vi "ROS_Dummy_Test.vi"() -> ()   [LabVIEW 2016]
uses:
  <userlib>/ROS for LabVIEW Software/ROS/Code/Console/Servers/ServerSubs/TopicDef.ctl
  <userlib>/ROS for LabVIEW Software/ROS/Code/SubVIs/_ROSDirection.ctl
  <userlib>/ROS for LabVIEW Software/ROS/MessageBuilding/std_msgs/subs/i32Scalar.vi
  <userlib>/ROS for LabVIEW Software/ROS/MessageBuilding/std_msgs/subs/boolScalar.vi
  <userlib>/ROS for LabVIEW Software/ROS/MessageParsing/std_msgs/subs/parse_string_scalar.vi
  <userlib>/ROS for LabVIEW Software/ROS/MessageParsing/std_msgs/subs/parse_float32_scalar.vi
  <userlib>/ROS for LabVIEW Software/ROS/MessageParsing/std_msgs/subs/parse_bool_scalar.vi
panel:
  in  "Run Lift":bool
  in  "Emergency STOP":bool
  out "lightStatus":bool
  out "uwbStatus":bool
  out "lidarBackStatus":bool
  out "liftStatus":bool
  out "UWB Position":cluster{"x":dbl, "y":dbl, "z":dbl}
  out "Lidar Back Dist":sgl
  out "Lift Done!":bool
  in  "TX2 Statemachine STATE":T1(ring)
  in  "STOP Program":bool
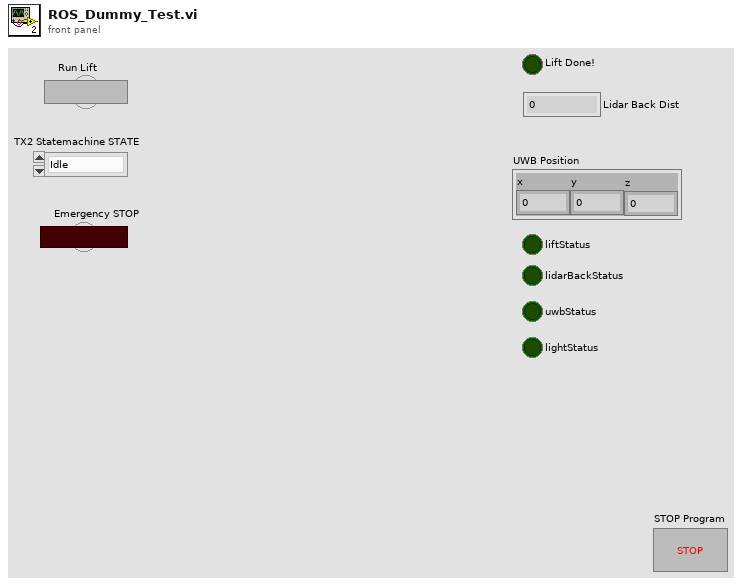
[diagram p1: front panel]
types:
  T1 = enum16{"Idle", "Moving", "2", "3", "4", "5", "6", "7", "Reversing"}
  T2 = typedef "TopicDef.ctl" = cluster{"Topic":string, "Type":string, "Action":T3, "Update (ms)":u16, "queue size":u16}
  T3 = typedef "_ROSDirection.ctl" = enum16{"Node", "Publisher", "Subscriber", "ServiceClient", "ServiceProvider"}
  T4 = typedef "_ROSControl.ctl" = cluster{"topic port":u16, "Node":string, "topic":string, "type":string, "node port":u16, "error ":errorcluster, "Direction":T3, "Update (ms)":u16, "FIFO size":u16}
  T5 = cluster{"status":cluster{"liftStatus":bool, "lidarBackStatus":bool, "uwbStatus":bool, "lightStatus":bool}}
  T6 = cluster{"liftStatus":bool, "lidarBackStatus":bool, "uwbStatus":bool, "lightStatus":bool}
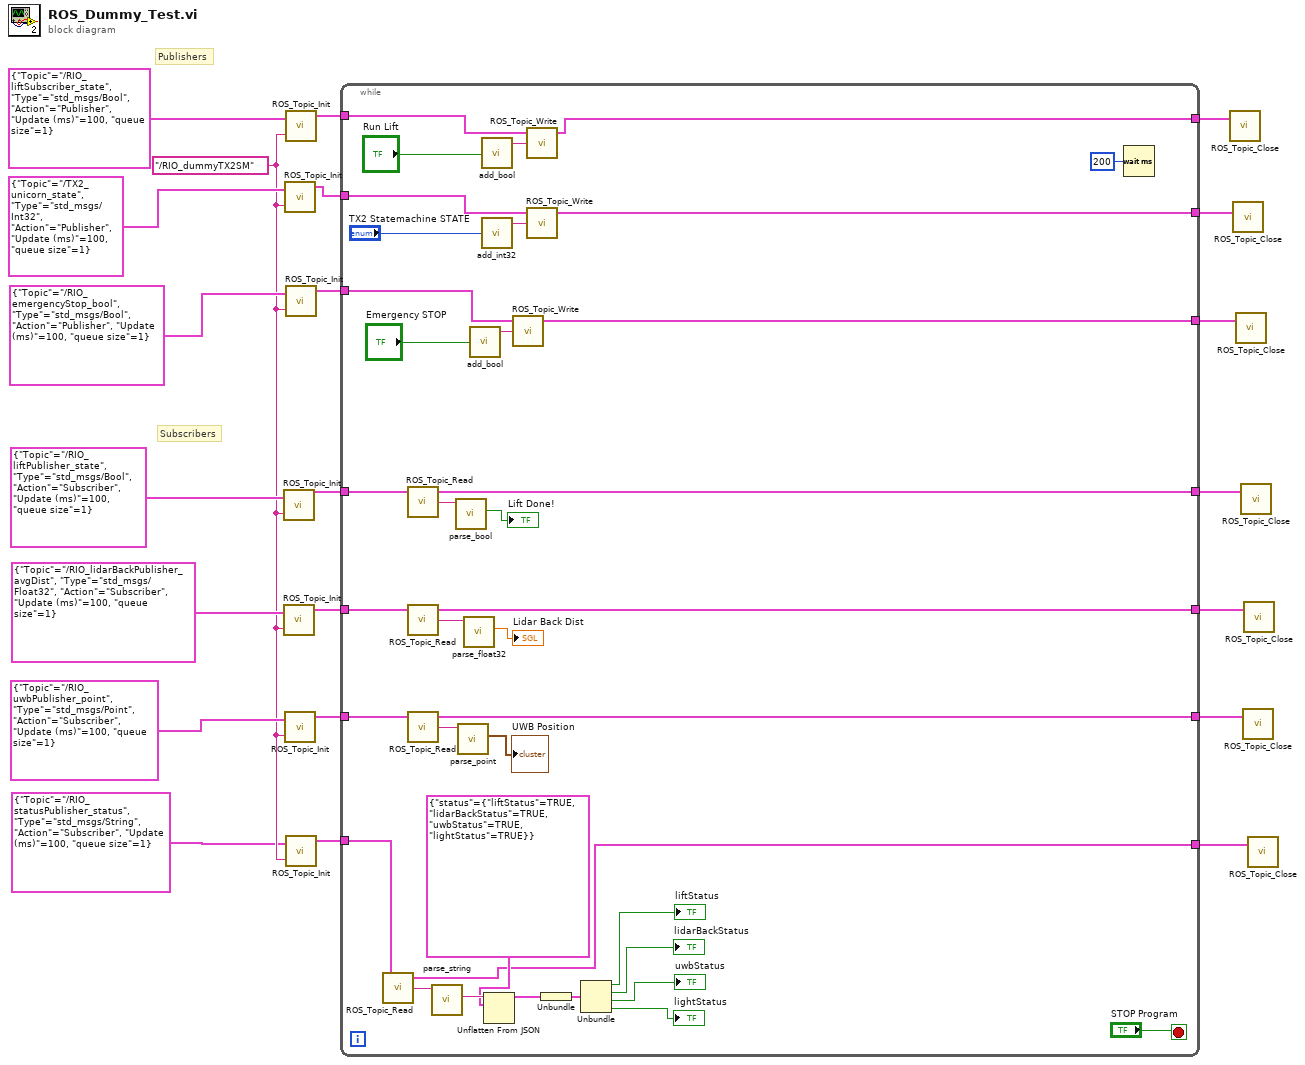
[diagram p0: block diagram]
diagram:
  w16 = "/RIO_dummyTX2SM" ("node")
  # "Publishers"
  # "Subscribers"
  n1 = call <userlib>:"ROS_Topic_Init.vi"("Definitions"=T2 {"Topic"="/RIO_liftPublisher_state", "Type"="std_msgs/Bool", "Action"=enum."Subscriber", "Update (ms)"=100, "queue size"=1}, "node"=w16) -> ("ROS out"=w8:T4)  [unwired: 1 in, 1 out]
  n2 = call <userlib>:"ROS_Topic_Init.vi"("Definitions"=T2 {"Topic"="/RIO_lidarBackPublisher_avgDist", "Type"="std_msgs/Float32", "Action"=enum."Subscriber", "Update (ms)"=100, "queue size"=1}, "node"=w16) -> ("ROS out"=w6:T4)  [unwired: 1 in, 1 out]
  n3 = call <userlib>:"ROS_Topic_Init.vi"("Definitions"=T2 {"Topic"="/TX2_unicorn_state", "Type"="std_msgs/Int32", "Action"=enum."Publisher", "Update (ms)"=100, "queue size"=1}, "node"=w16) -> ("ROS out"=w12:T4)  [unwired: 1 in, 1 out]
  n4 = call <userlib>:"ROS_Topic_Init.vi"("Definitions"=T2 {"Topic"="/RIO_uwbPublisher_point", "Type"="std_msgs/Point", "Action"=enum."Subscriber", "Update (ms)"=100, "queue size"=1}, "node"=w16) -> ("ROS out"=w4:T4)  [unwired: 1 in, 1 out]
  n5 = call <userlib>:"ROS_Topic_Init.vi"("Definitions"=T2 {"Topic"="/RIO_liftSubscriber_state", "Type"="std_msgs/Bool", "Action"=enum."Publisher", "Update (ms)"=100, "queue size"=1}, "node"=w16) -> ("ROS out"=w14:T4)  [unwired: 1 in, 1 out]
  n6 = call <userlib>:"ROS_Topic_Init.vi"("Definitions"=T2 {"Topic"="/RIO_emergencyStop_bool", "Type"="std_msgs/Bool", "Action"=enum."Publisher", "Update (ms)"=100, "queue size"=1}, "node"=w16) -> ("ROS out"=w10:T4)  [unwired: 1 in, 1 out]
  n7 = call <userlib>:"ROS_Topic_Init.vi"("Definitions"=T2 {"Topic"="/RIO_statusPublisher_status", "Type"="std_msgs/String", "Action"=enum."Subscriber", "Update (ms)"=100, "queue size"=1}, "node"=w16) -> ("ROS out"=w2:T4)  [unwired: 1 in, 1 out]
  n8 = while {
    tunnel: w14 -> [w58]
    tunnel: [w57] -> w13
    tunnel: w12 -> [w56]
    tunnel: [w54] -> w11
    tunnel: w10 -> [w51]
    tunnel: [w50] -> w9
    tunnel: w8 -> [w47]
    tunnel: [w46] -> w7
    tunnel: w6 -> [w45]
    tunnel: [w42] -> w5
    tunnel: w4 -> [w41]
    tunnel: [w38] -> w3
    tunnel: w2 -> [w37]
    tunnel: [w27] -> w1
    stop <- "STOP Program" stop-if-true
    n9 = call <userlib>:"ROS_Topic_Read.vi"("ROS in"=w37) -> ("Reply"=w36:string, "ROS out"=w27:T4)  [unwired: 2 in, 1 out]
    n10 = call <userlib>:"ROS_Topic_Read.vi"("ROS in"=w47) -> ("Reply"=w49:string, "ROS out"=w46:T4)  [unwired: 2 in, 1 out]
    n11 = call <userlib>:"ROS_Topic_Read.vi"("ROS in"=w45) -> ("Reply"=w44:string, "ROS out"=w42:T4)  [unwired: 2 in, 1 out]
    n12 = call <userlib>:"ROS_Topic_Read.vi"("ROS in"=w41) -> ("Reply"=w40:string, "ROS out"=w38:T4)  [unwired: 2 in, 1 out]
    n13 = call-poly <userlib>:"parse_string.vi"("msg in"=w36) -> ("string"=w35:string)  [unwired: 4 in, 2 out]
    n14 = call-poly <userlib>:"parse_bool.vi"("msg in"=w49) -> ("bool"=→"Lift Done!":bool)  [unwired: 4 in, 2 out]
    n15 = call <userlib>:"parse_point.vi"("msg in"=w40) -> ("Point"=→"UWB Position":cluster{"x":dbl, "y":dbl, "z":dbl})  [unwired: 4 in, 2 out]
    n16 = call-poly <userlib>:"parse_float32.vi"("msg in"=w44) -> ("number"=→"Lidar Back Dist":sgl)  [unwired: 4 in, 2 out]
    n17 = call-poly <userlib>:"add_bool.vi"("Boolean"="Emergency STOP") -> ("msg out"=w52:string)  [unwired: 4 in]
    n18 = call-poly <userlib>:"add_bool.vi"("Boolean"="Run Lift") -> ("msg out"=w24:string)  [unwired: 4 in]
    n19 = call-poly <userlib>:"add_int32.vi"("Numeric"="TX2 Statemachine STATE") -> ("msg out"=w55:string)  [unwired: 4 in]
    n20 = Unflatten From JSON(JSON string=w35, type and defaults=T5 {"status"={"liftStatus"=TRUE, "lidarBackStatus"=TRUE, "uwbStatus"=TRUE, "lightStatus"=TRUE}}) -> (value=w34:T5)  [unwired: 5 in, 1 out]
    n21 = call <userlib>:"ROS_Topic_Write.vi"("Msg in"=w52, "ROS in"=w51) -> ("ROS out"=w50:T4)  [unwired: 2 in, 1 out]
    n22 = call <userlib>:"ROS_Topic_Write.vi"("Msg in"=w24, "ROS in"=w58) -> ("ROS out"=w57:T4)  [unwired: 2 in, 1 out]
    n23 = call <userlib>:"ROS_Topic_Write.vi"("Msg in"=w55, "ROS in"=w56) -> ("ROS out"=w54:T4)  [unwired: 2 in, 1 out]
    n24 = Unbundle(w34) -> ("status"=w32:T6)
    n25 = Unbundle(w32) -> ("liftStatus"=→"liftStatus":bool, "lidarBackStatus"=→"lidarBackStatus":bool, "uwbStatus"=→"uwbStatus":bool, "lightStatus"=→"lightStatus":bool)
    n26 = Wait (ms)(milliseconds to wait=u32 200) -> ()  [unwired: 1 out]
  }
  n27 = call <userlib>:"ROS_Topic_Close.vi"("ROS in"=w13) -> ()  [unwired: 3 in, 1 out]
  n28 = call <userlib>:"ROS_Topic_Close.vi"("ROS in"=w11) -> ()  [unwired: 3 in, 1 out]
  n29 = call <userlib>:"ROS_Topic_Close.vi"("ROS in"=w9) -> ()  [unwired: 3 in, 1 out]
  n30 = call <userlib>:"ROS_Topic_Close.vi"("ROS in"=w7) -> ()  [unwired: 3 in, 1 out]
  n31 = call <userlib>:"ROS_Topic_Close.vi"("ROS in"=w3) -> ()  [unwired: 3 in, 1 out]
  n32 = call <userlib>:"ROS_Topic_Close.vi"("ROS in"=w5) -> ()  [unwired: 3 in, 1 out]
  n33 = call <userlib>:"ROS_Topic_Close.vi"("ROS in"=w1) -> ()  [unwired: 3 in, 1 out]
